vi "viewStatus.vi"(8 "error in (no error)":errorcluster, 10 "return elements? (F)":bool, 11 "MissionQueue in":refnum<class "MissionQueue.lvclass">) -> (0 "error out":errorcluster, 1 "Queue length":i32, 2 "Is empty?":bool, 3 "MissionQueue out":refnum<class "MissionQueue.lvclass">, 4 "elements":refnum<class "GenericMission.lvclass">[](array[class]))   [LabVIEW 2011, in "MissionQueue.lvclass"]
doc: "Views the mission queue and returns how many elements the queue contains and whether or not it is empty."
uses:
  MissionQueue.lvclass
  Missions/GenericMission/GenericMission.lvclass
  MissionQueue.lvclass/MissionQueue.ctl
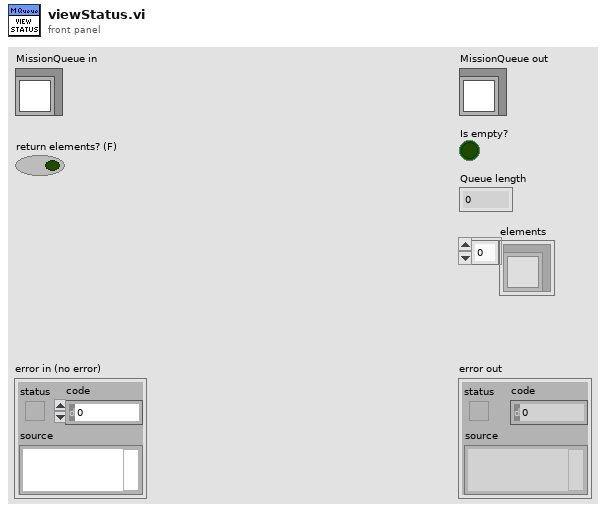
[diagram p1: front panel]
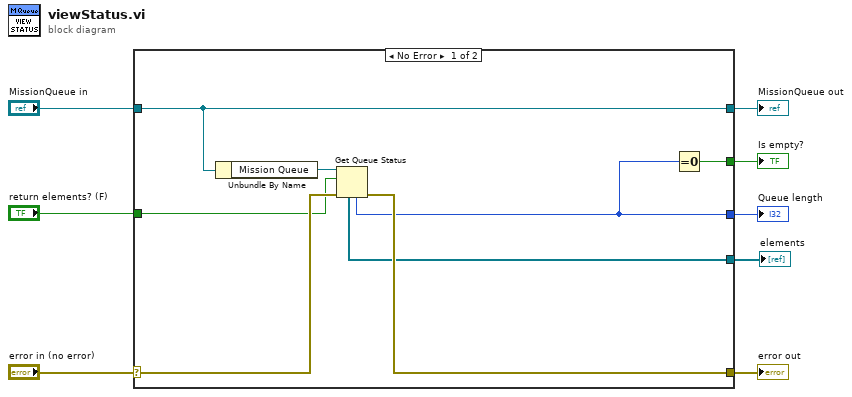
[diagram p0: block diagram]
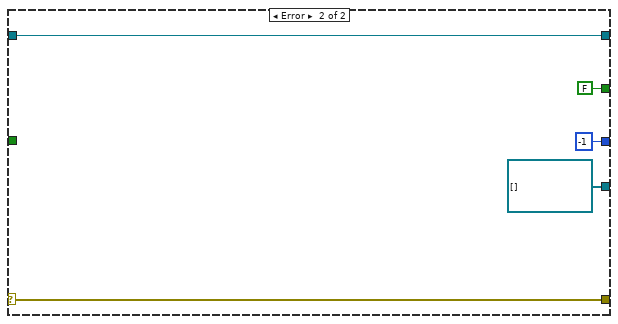
[diagram p2: hidden frame]
diagram:
  n1 = case shown="No Error" "error in (no error)" {
    selector: "error in (no error)" -> [w14 w21]
    tunnel: [w13 w21] -> w7
    tunnel: [w16 w20] -> w5
    tunnel: "MissionQueue in" -> [w16 w20]
    tunnel: [w12 FALSE] -> w4
    tunnel: [w11 -1 ("# elements in queue")] -> w3
    tunnel: [w10 refnum<class "GenericMission.lvclass">[] [] ("elements")] -> w2
    tunnel: "return elements? (F)" -> [w9 _]
    frame No Error {
      n2 = Unbundle By Name(w16) -> ("Mission Queue"=w15:refnum<queue>)
      n3 = Get Queue Status(queue=w15, return elements? (F)=w9, error in (no error)=w14) -> (error out=w13:errorcluster, # elements in queue=w11:i32, elements=w10:refnum<class "GenericMission.lvclass">[])  [unwired: 5 out]
      n4 = Equal To 0?(x=w11) -> (x = 0?=w12:bool)
    }
    frame Error {
    }
  }
  "error out" <- w7
  "MissionQueue out" <- w5
  "Is empty?" <- w4
  "Queue length" <- w3
  "elements" <- w2
